vi "readInAoXML.vi"(8 "error in (no error)":errorcluster, 10 "NativeXML in":refnum<class "NativeXML.lvclass">, 11 "deviceDataBase in":refnum<class "deviceDataBase.lvclass">) -> (0 "error out":errorcluster, 1 "device.lvclass out":refnum<class "device.lvclass">, 3 "deviceDataBase out":refnum<class "deviceDataBase.lvclass">)   [LabVIEW 2009, in "Tools.lvlib" / "DatabaseHelpers.lvlib" / "deviceDataBase.lvclass"]
uses:
  deviceDataBase.lvclass
  NativeXML/NativeXML.lvclass
  Database Objects/device/device.lvclass
  Database Objects/device/AnalogDevice/AnalogDevice.lvclass
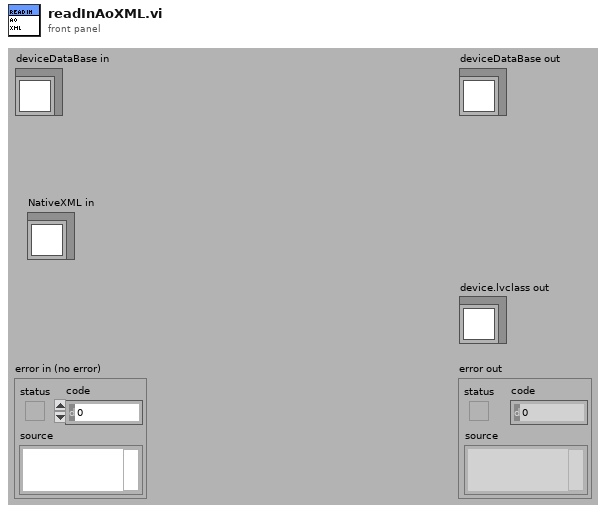
[diagram p1: front panel]
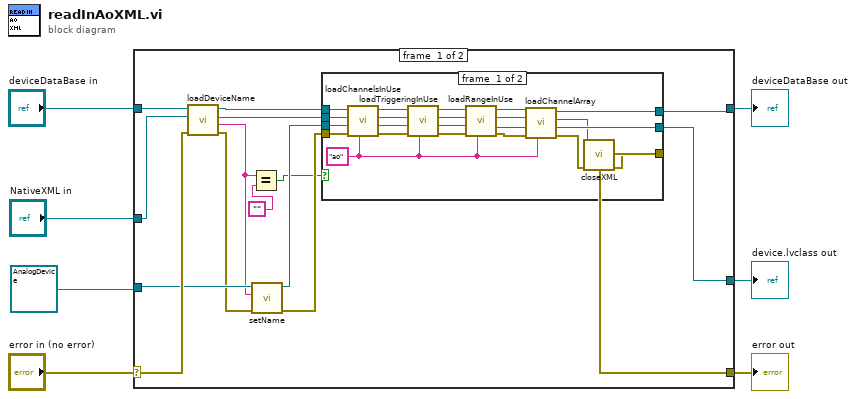
[diagram p0: block diagram]
diagram:
  n1 = case shown="No Error" "error in (no error)" {
    selector: "error in (no error)" -> [w21 w49]
    tunnel: [w13 w49] -> w6
    tunnel: [w12 w48] -> w4
    tunnel: "deviceDataBase in" -> [w22 w48]
    tunnel: "NativeXML in" -> [w20 _]
    tunnel: refnum<class "AnalogDevice.lvclass"> refnum ("Tools.lvlib:DatabaseHelpers.lvlib:AnalogDevice.lvclass") -> [w19 _]
    tunnel: [w8 _] -> w1
    frame #0 {
      n2 = call "loadDeviceName.vi"("error in (no error)"=w21, "NativeXML in"=w20, "deviceDataBase in"=w22) -> ("error out"=w18:errorcluster, "deviceName"=w9:string, "NativeXML out"=w15:refnum<class "NativeXML.lvclass">, "deviceDataBase out"=w17:refnum<class "deviceDataBase.lvclass">)  [unwired: 5 in]
      n3 = Equal?(x=w9, y="") -> (x = y?=w11:bool)
      n4 = call "setName.vi"("error in (no error)"=w18, "name"=w9, "device.lvclass in"=w19) -> ("error out"=w16:errorcluster, "device.lvclass out"=w14:refnum<class "AnalogDevice.lvclass">)  [unwired: 7 in]
      n5 = case shown="False" w11 {
        tunnel: w17 -> [w44 w47]
        tunnel: w16 -> [w43 w45]
        tunnel: w15 -> [w42 _]
        tunnel: w14 -> [w41 w46]
        tunnel: [w23 w45] -> w13
        tunnel: [w28 w46] -> w8
        tunnel: [w27 w47] -> w12
        frame #0 {
          w26 = "ao"
          n6 = call "loadChannelsInUse.vi"("type"=w26, "error in (no error)"=w43, "device.lvclass"=w41, "NativeXML in"=w42, "deviceDataBase in"=w44) -> ("error out"=w40:errorcluster, "device.lvclass out"=w37:refnum<class "device.lvclass">, "NativeXML out"=w38:refnum<class "NativeXML.lvclass">, "deviceDataBase out"=w39:refnum<class "deviceDataBase.lvclass">)  [unwired: 3 in]
          n7 = call "loadTriggeringInUse.vi"("type"=w26, "error in (no error)"=w40, "device.lvclass"=w37, "NativeXML in"=w38, "deviceDataBase in"=w39) -> ("error out"=w33:errorcluster, "device.lvclass out"=w34:refnum<class "device.lvclass">, "NativeXML out"=w35:refnum<class "NativeXML.lvclass">, "deviceDataBase out"=w36:refnum<class "deviceDataBase.lvclass">)  [unwired: 3 in]
          n8 = call "loadRangeInUse.vi"("type"=w26, "error in (no error)"=w33, "device.lvclass"=w34, "NativeXML in"=w35, "deviceDataBase in"=w36) -> ("error out"=w31:errorcluster, "device.lvclass out"=w29:refnum<class "device.lvclass">, "NativeXML out"=w30:refnum<class "NativeXML.lvclass">, "deviceDataBase out"=w32:refnum<class "deviceDataBase.lvclass">)  [unwired: 3 in]
          n9 = call "loadChannelArray.vi"("type"=w26, "error in (no error)"=w31, "device.lvclass"=w29, "NativeXML in"=w30, "deviceDataBase in"=w32) -> ("error out"=w25:errorcluster, "device.lvclass out"=w28:refnum<class "device.lvclass">, "NativeXML out"=w24:refnum<class "NativeXML.lvclass">, "deviceDataBase out"=w27:refnum<class "deviceDataBase.lvclass">)  [unwired: 3 in]
          n10 = call "closeXML.vi"("error in (no error)"=w25, "NativeXML in"=w24) -> ("error out"=w23:errorcluster)  [unwired: 9 in]
        }
        frame #1 {
        }
      }
    }
    frame #1 {
    }
  }
  "error out" <- w6
  "deviceDataBase out" <- w4
  "device.lvclass out" <- w1
